vi "daq_example_ai.vi"() -> ()   [LabVIEW 2015]
uses:
  <vilib>/DAQmx/read.llb/DAQmx Read (Analog 1D Wfm NChan NSamp).vi
  <vilib>/DAQmx/create/channels.llb/DAQmx Create Channel (AI-Voltage-Basic).vi
  <vilib>/DAQmx/configure/timing.llb/DAQmx Timing (Sample Clock).vi
  <vilib>/DAQmx/miscellaneous.llb/DAQmx Fill In Error Info.vi
panel:
  in  "Start":bool
  in  "Stop":bool
  out "Waveform Chart":waveform(dbl)[](graph)
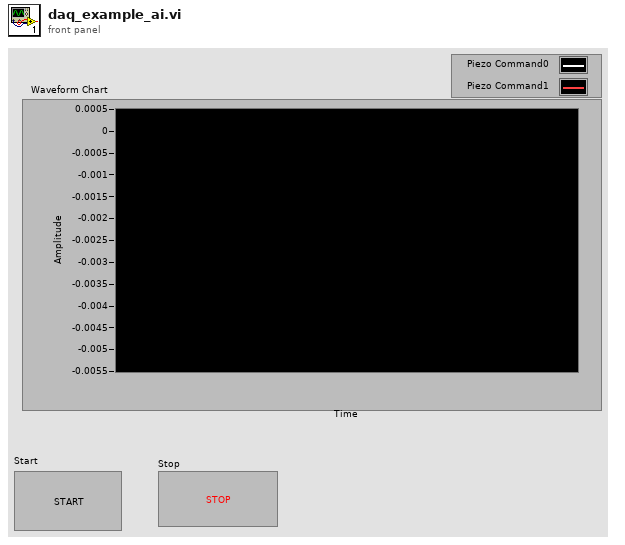
[diagram p1: front panel]
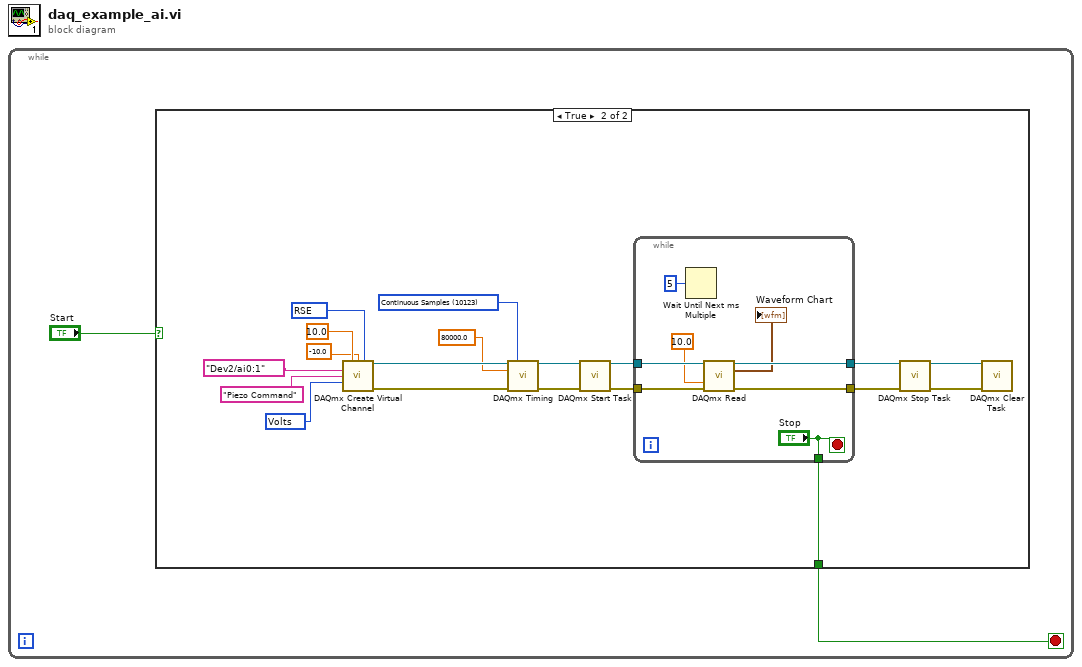
[diagram p0: block diagram]
diagram:
  n1 = while {
    stop <- w1 stop-if-true
    n2 = case shown="True" "Start" {
      tunnel: [_ w11] -> w1
      frame False {
      }
      frame True {
        w7 = 10083 items=["default"=-1, "RSE"=10083, "NRSE"=10078, "Differential"=10106, "Pseudodifferential"=12529] ("input terminal configuration")
        w8 = 10123 items=["Finite Samples"=10178, "Continuous Samples"=10123] ("sample mode")
        w9 = 10348 items=["Volts"=10348, "From Custom Scale"=10065] ("units")
        n3 = call-poly <vilib>:"DAQmx Create Virtual Channel.vi"("maximum value"=10.0, "minimum value"=-10.0, "input terminal configuration"=w7, "physical channels"=tag "Dev2/ai0:1" ("DAQmx Physical Channel"), "name to assign"="Piezo Command", "units"=w9) -> ("task out"=w16:refnum<k21>, "error out"=w17:errorcluster)  [unwired: 8 in]
        n4 = call-poly <vilib>:"DAQmx Timing.vi"("task/channels in"=w16, "sample mode"=w8, "rate"=80000.0, "error in"=w17) -> ("task out"=w6:refnum<k21>, "error out"=w5:errorcluster)  [unwired: 10 in]
        n5 = call <vilib>:"DAQmx Start Task.vi"("task/channels in"=w6, "error in"=w5) -> ("task out"=w3:refnum<k21>, "error out"=w4:errorcluster)  [unwired: 12 in]
        n6 = while {
          tunnel: ["Stop"] -> w11
          tunnel: w3 -> [w26]
          tunnel: [w29] -> w20
          tunnel: w4 -> [w27]
          tunnel: [w28] -> w19
          stop <- "Stop" stop-if-true
          n7 = Wait Until Next ms Multiple(millisecond multiple=u32 5) -> ()  [unwired: 1 out]
          n8 = call-poly <vilib>:"DAQmx Read.vi"("task/channels in"=w26, "timeout"=10.0, "error in"=w27) -> ("task out"=w29:refnum<k21>, "data"=→"Waveform Chart":waveform(dbl)[], "error out"=w28:errorcluster)  [unwired: 10 in]
        }
        n9 = call <vilib>:"DAQmx Stop Task.vi"("task/channels in"=w20, "error in"=w19) -> ("task out"=w21:refnum<k21>, "error out"=w18:errorcluster)  [unwired: 12 in]
        n10 = call <vilib>:"DAQmx Clear Task.vi"("task in"=w21, "error in"=w18) -> ()  [unwired: 13 in, 1 out]
      }
    }
  }
